vi "ClearWorkingDirectory.vi"(8 "error in":errorcluster, 11 "Working Path":path) -> (0 "error out":errorcluster, 3 "Working Path Out":path)   [LabVIEW 2024]
uses:
  <userlib>/_OpenG.lib/file/file.llb/openg_file.lvlib
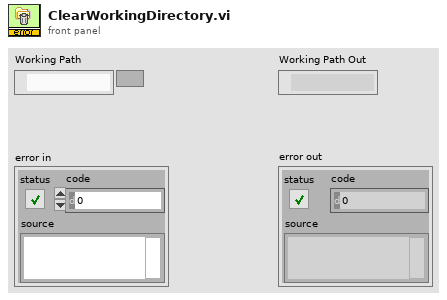
[diagram p1: front panel]
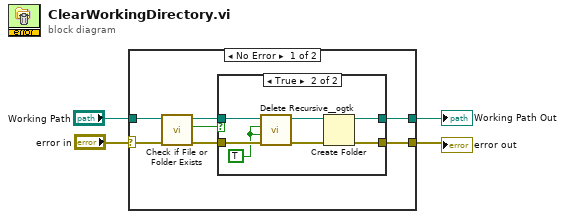
[diagram p0: block diagram]
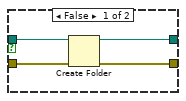
[diagram p2: hidden frame]
diagram:
  n1 = case shown="No Error" "error in" {
    selector: "error in" -> [w9 w24]
    tunnel: "Working Path" -> [w8 w23]
    tunnel: [w11 w23] -> w3
    tunnel: [w10 w24] -> w2
    frame No Error {
      n2 = call <vilib>:"Check if File or Folder Exists.vi"("error in (no error)"=w9, "path"=w8) -> ("error out"=w6:errorcluster, "file or folder exists?"=w5:bool, "dup path"=w7:path)  [unwired: 7 in]
      n3 = case shown="True" w5 {
        tunnel: w6 -> [w15 w21]
        tunnel: w7 -> [w14 w22]
        tunnel: [w12 w17] -> w11
        tunnel: [w13 w18] -> w10
        frame False {
          n4 = Create Folder(path (use dialog)=w14, error in=w15) -> (created path=w12:path, error out=w13:errorcluster)  [unwired: 1 in, 1 out]
        }
        frame True {
          w16 = TRUE ("Ignore Read-Only? (FALSE)")
          n5 = call <userlib>:"Delete Recursive__ogtk.vi"("error in (no error)"=w21, "Ignore Read-Only? (FALSE)"=w16, "Recursive? (FALSE)"=w16, "Path"=w22) -> ("error out"=w19:errorcluster, "dup Path"=w20:path)  [unwired: 6 in]
          n6 = Create Folder(path (use dialog)=w20, error in=w19) -> (created path=w17:path, error out=w18:errorcluster)  [unwired: 1 in, 1 out]
        }
      }
    }
    frame Error {
    }
  }
  "Working Path Out" <- w3
  "error out" <- w2
